vi "xml_tree.vi"() -> ()   [LabVIEW 2013]
uses:
  <vilib>/xml/Load XML File.vi
  <vilib>/xml/NI_XML.lvlib
  <resource>/objmgr/DOMUserDefRef.rc
panel:
  out "Active Item:Indent Level":i32
  in  "stop":bool
  out "current tree level":i32
  in  "Tree":string(tree)
  out "parse errors":string
  out "Node Value":string
  out "Parent Node Name":string
  out "Child Node Name":string
  out "XML":string
  in  "xml file":path
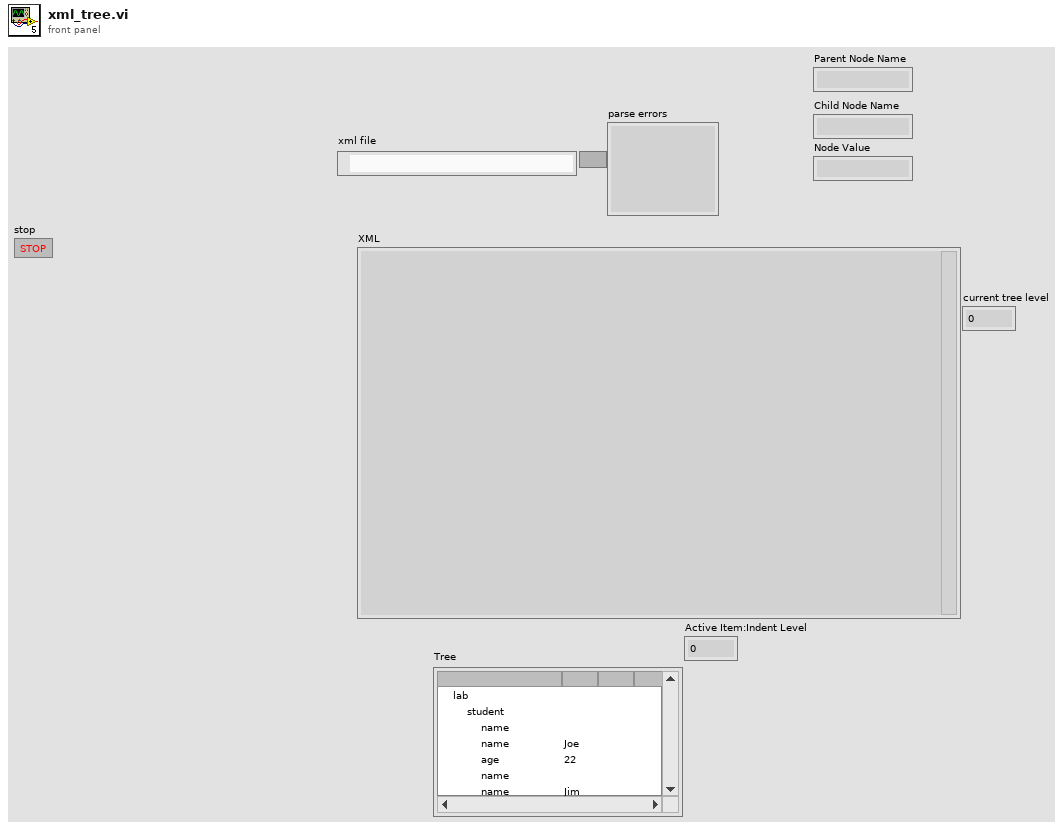
[diagram p1: front panel]
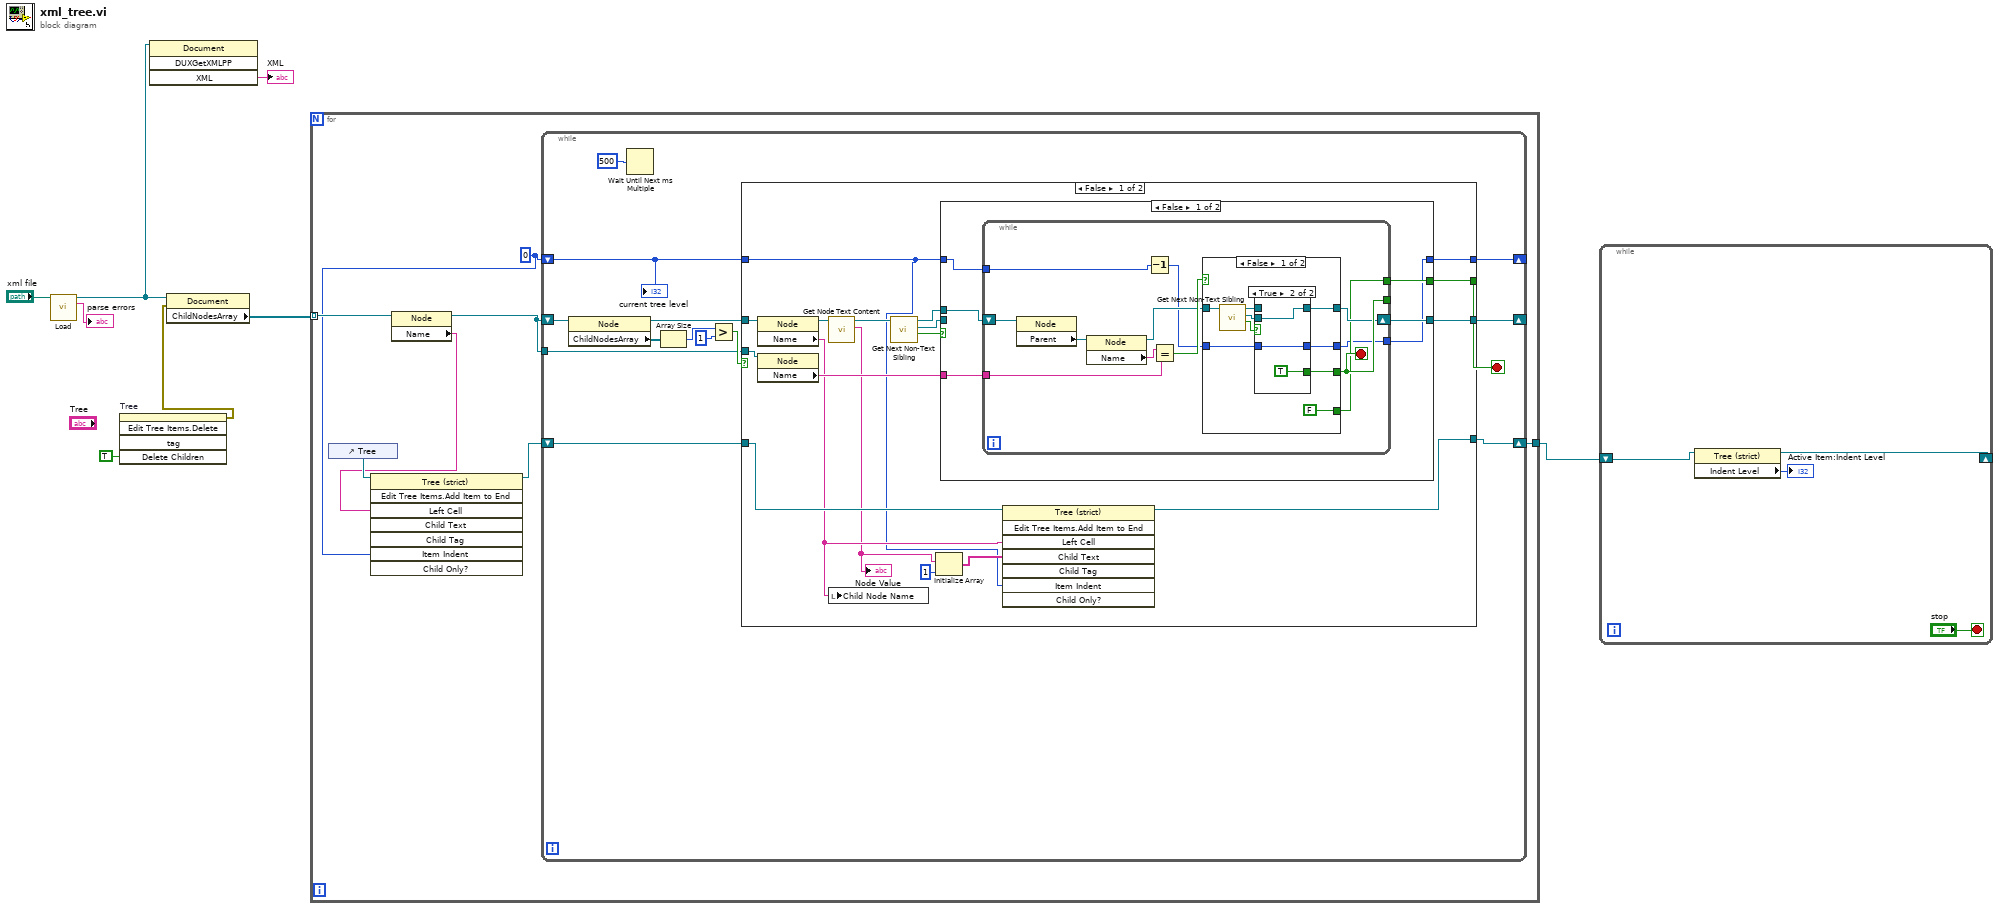
[diagram p0: block diagram]
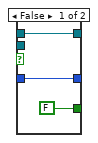
[diagram p2: hidden frame]
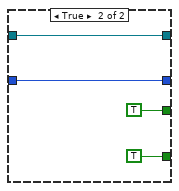
[diagram p3: hidden frame]
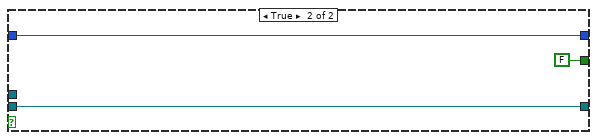
[diagram p4: hidden frame]
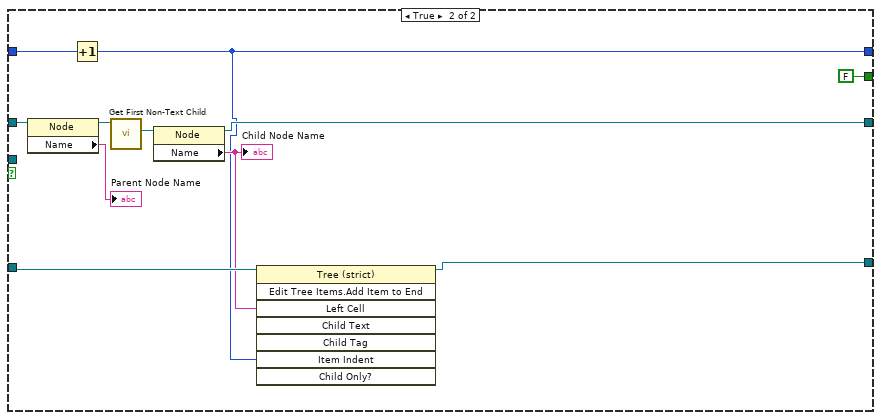
[diagram p5: hidden frame]
diagram:
  n1 = call-poly <vilib>:"Load.vi"("path to XML document"="xml file") -> ("DOM document out"=w6:refnum<k20>, "parse errors"=→"parse errors":string)  [unwired: 12 in, 1 out]
  n2 = invoke on="Tree" class="Tree (strict)" method="Edit Tree Items.Delete"("Delete Children"=TRUE ("Delete Children?")) -> (error out=w2:errorcluster)  [unwired: 4 in, 4 out]
  n3 = invoke class="Document" method="DUXGetXMLPP"(reference=w6) -> ("XML"=→"XML":string)  [unwired: 3 in, 3 out]
  n4 = property class="Document"(reference=w6, error in=w2) -> ("ChildNodesArray"=w7:refnum<k20>[])  [unwired: 2 out]
  n5 = for {
    tunnel: w7 -> [w15] mode=indexing
    tunnel: [w9] -> w1
    w10 = 0 ("x")
    n6 = control-ref of="Tree"() -> (w13:refnum<vi>)
    n7 = property class="Node"(reference=w15) -> (reference out=w14:refnum<k20>, "Name"=w11:string)  [unwired: 1 in, 1 out]
    n8 = invoke class="Tree (strict)" method="Edit Tree Items.Add Item to End"(reference=w13, "Left Cell"=w11, "Item Indent"=w10) -> (reference out=w12:refnum<vi>)  [unwired: 5 in, 7 out]
    n9 = while {
      shift-right: [w29] -> _
      shift-left: w14 -> [w19]
      tunnel: w14 -> [w22]
      shift-right: [w20] -> _
      shift-left: w10 -> [w18]
      shift-right: [w16] -> w9
      shift-left: w12 -> [w17]
      stop <- w23 stop-if-true
      n10 = property class="Node"(reference=w19) -> (reference out=w24:refnum<k20>, "ChildNodesArray"=w28:refnum<k20>[])  [unwired: 1 in, 1 out]
      n11 = Wait Until Next ms Multiple(millisecond multiple=u32 500) -> ()  [unwired: 1 out]
      n12 = Array Size(array=w28) -> (size(s)=w27:i32)
      n13 = Greater?(x=w27, y=1) -> (0:w25:bool)
      n14 = case shown="False" w25 {
        tunnel: [w43 w98] -> w29
        tunnel: w24 -> [w47 w95]
        tunnel: [w40 FALSE] -> w23
        tunnel: w22 -> [w39 _]
        tunnel: w18 -> [w30 w93]
        tunnel: [w37 w88] -> w20
        tunnel: w17 -> [w36 w91]
        tunnel: [w35 w90] -> w16
        frame False {
          n15 = property class="Node"(reference=w47) -> (reference out=w46:refnum<k20>, "Name"=w34:string)  [unwired: 1 in, 1 out]
          n16 = property class="Node"(reference=w39) -> ("Name"=w38:string)  [unwired: 1 in, 2 out]
          n17 = call <vilib>:"Get Node Text Content.vi"("node in"=w46) -> ("node text"=w32:string, "node out"=w45:refnum<k20>)  [unwired: 8 in, 1 out]
          "Node Value" <- w32
          n18 = local write "Child Node Name"(w34) -> ()
          n19 = call <vilib>:"Get Next Non-Text Sibling.vi"("node in"=w45) -> ("found sibling node?"=w44:bool, "sibling node"=w42:refnum<k20>, "node out"=w41:refnum<k20>)  [unwired: 7 in, 1 out]
          n20 = Initialize Array(w32, 1 ("dimension size")) -> (w31:string[])
          n21 = case shown="False" w44 {
            tunnel: [w53 w87] -> w43
            tunnel: w42 -> [_ w87]
            tunnel: w41 -> [w52 _]
            tunnel: [w51 FALSE] -> w40
            tunnel: w38 -> [w50 _]
            tunnel: [w48 w85] -> w37
            tunnel: w30 -> [w49 w85]
            frame False {
              n22 = while {
                shift-right: [w63] -> w53
                shift-left: w52 -> [w64]
                tunnel: [w65] -> _
                tunnel: [w61] -> w51
                tunnel: w50 -> [w57]
                tunnel: w49 -> [w54]
                tunnel: [w56] -> w48
                stop <- w65 stop-if-true
                n23 = property class="Node"(reference=w64) -> ("Parent"=w60:refnum<k20>)  [unwired: 1 in, 2 out]
                n24 = property class="Node"(reference=w60) -> (reference out=w59:refnum<k20>, "Name"=w58:string)  [unwired: 1 in, 1 out]
                n25 = Decrement(x=w54) -> (x-1=w55:i32)
                n26 = Equal?(x=w58, y=w57) -> (x = y?=w62:bool)
                n27 = case shown="False" w62 {
                  tunnel: [w74 TRUE] -> w65
                  tunnel: [w73 w83] -> w63
                  tunnel: w59 -> [w69 w83]
                  tunnel: [FALSE TRUE] -> w61
                  tunnel: w55 -> [w67 w81]
                  tunnel: [w66 w81] -> w56
                  frame False {
                    n28 = call <vilib>:"Get Next Non-Text Sibling.vi"("node in"=w69) -> ("found sibling node?"=w70:bool, "sibling node"=w72:refnum<k20>, "node out"=w71:refnum<k20>)  [unwired: 7 in, 1 out]
                    n29 = case shown="True" w70 {
                      tunnel: [w77 w80] -> w73
                      tunnel: w72 -> [_ w80]
                      tunnel: w71 -> [w77 _]
                      tunnel: [FALSE TRUE] -> w74
                      tunnel: w67 -> [w75 w78]
                      tunnel: [w75 w78] -> w66
                      frame False {
                      }
                      frame True {
                      }
                    }
                  }
                  frame True {
                  }
                }
              }
            }
            frame True {
            }
          }
          n30 = invoke class="Tree (strict)" method="Edit Tree Items.Add Item to End"(reference=w36, "Left Cell"=w34, "Child Text"=w31, "Item Indent"=w30) -> (reference out=w35:refnum<vi>)  [unwired: 4 in, 7 out]
        }
        frame True {
          n31 = property class="Node"(reference=w95) -> (reference out=w96:refnum<k20>, "Name"=→"Parent Node Name":string)  [unwired: 1 in, 1 out]
          n32 = Increment(x=w93) -> (x+1=w88:i32)
          n33 = call <vilib>:"Get First Non-Text Child.vi"("node in"=w96) -> ("child node"=w97:refnum<k20>)  [unwired: 7 in, 3 out]
          n34 = property class="Node"(reference=w97) -> (reference out=w98:refnum<k20>, "Name"=w89:string)  [unwired: 1 in, 1 out]
          "Child Node Name" <- w89
          n35 = invoke class="Tree (strict)" method="Edit Tree Items.Add Item to End"(reference=w91, "Left Cell"=w89, "Item Indent"=w88) -> (reference out=w90:refnum<vi>)  [unwired: 5 in, 7 out]
        }
      }
      "current tree level" <- w18
    }
  }
  n36 = while {
    shift-right: [w99] -> _
    shift-left: w1 -> [w101]
    stop <- "stop" stop-if-true
    n37 = property class="Tree (strict)"(reference=w101) -> (reference out=w99:refnum<vi>, "Indent Level"=→"Active Item:Indent Level":i32)  [unwired: 1 in, 1 out]
  }
